vi "GUI_Syringe_Pump.vi"() -> ()   [LabVIEW 2020]
uses:
  <vilib>/Instr/_visa.llb/VISA Configure Serial Port (Instr).vi
panel:
  in  "Reset4":bool
  in  "Reset3":bool
  in  "Reset2":bool
  out "Remains4":string
  out "Remains3":string
  out "Remains2":string
  out "Dispensed4":string
  out "Dispensed3":string
  out "Dispensed2":string
  in  "Pump4\nStart/Stop":bool
  in  "Pump3\nStart/Stop":bool
  in  "Pump2\nStart/Stop":bool
  out "Diameter4 (mm)":dbl
  in  "dia4 (mm)":dbl=0.1 caption="Set Diameter (mm)" min=0.1 max=50.0
  in  "Syringe Selection4":string(combo)="CUS"
  out "Min rate4":dbl caption="Min rate" format="%#_4g"
  out "Max rate4":dbl format="%#_4g"
  in  "Direction4":string(combo)="inf"
  in  "Target Vol4":dbl caption="Target Vol (ul)"
  in  "Units4":string(combo)="mm"
  in  "Set rate4":dbl format="%#_4g"
  out "Diameter3 (mm)":dbl
  in  "dia3 (mm)":dbl=0.1 caption="Set Diameter (mm)" min=0.1 max=50.0
  in  "Syringe Selection3":string(combo)="CUS"
  out "Min rate3":dbl caption="Min rate" format="%#_4g"
  out "Max rate3":dbl format="%#_4g"
  in  "Direction3":string(combo)="inf"
  in  "Target Vol3":dbl caption="Target Vol (ul)"
  in  "Units3":string(combo)="mm"
  in  "Set rate3":dbl format="%#_4g"
  out "Diameter2 (mm)":dbl
  in  "dia2 (mm)":dbl=0.1 caption="Set Diameter (mm)" min=0.1 max=50.0
  in  "Syringe Selection2":string(combo)="BDP1MM"
  out "Min rate2":dbl caption="Min rate" format="%#_4g"
  out "Max rate2":dbl format="%#_4g"
  in  "Direction2":string(combo)="inf"
  in  "Target Vol2":dbl=1234.0 caption="Target Vol (ul)"
  in  "Units2":string(combo)="uh"
  in  "Set rate2":dbl=1000.0 format="%#_4g"
  out "Diameter1 (mm)":dbl
  in  "Syringe Selection1":string(combo)="BDP1MM"
  out "Remains1":string
  in  "Reset1":bool
  out "Dispensed1":string
  out "Baud Rate":string
  in  "Communication\nOn/Off":bool=TRUE
  in  "Pump1\nStart/Stop":bool
  out "Min rate1":dbl caption="Min rate" format="%#_4g"
  out "Max rate1":dbl format="%#_4g"
  in  "Send1":bool
  in  "Direction1":string(combo)="inf"
  in  "Target Vol1":dbl=1000.0 caption="Target Vol (ul)"
  in  "Units1":string(combo)="uh"
  in  "Set rate1":dbl=123.0 format="%#_4g"
  in  "dia1 (mm)":dbl=0.1 caption="Set Diameter (mm)" min=0.1 max=50.0
  in  "COM port number":refnum<visa-resource-name>
  # "Communication Setting"
  # "Cockpit"
  # "Pump1"
  # "Pump3"
  # "Pump4"
  # "Pump2"
  # "[Pump1] Syringe Setting"
  # "[Pump2] Syringe Setting"
  # "[Pump3] Syringe Setting"
  # "[Pump4] Syringe Setting"
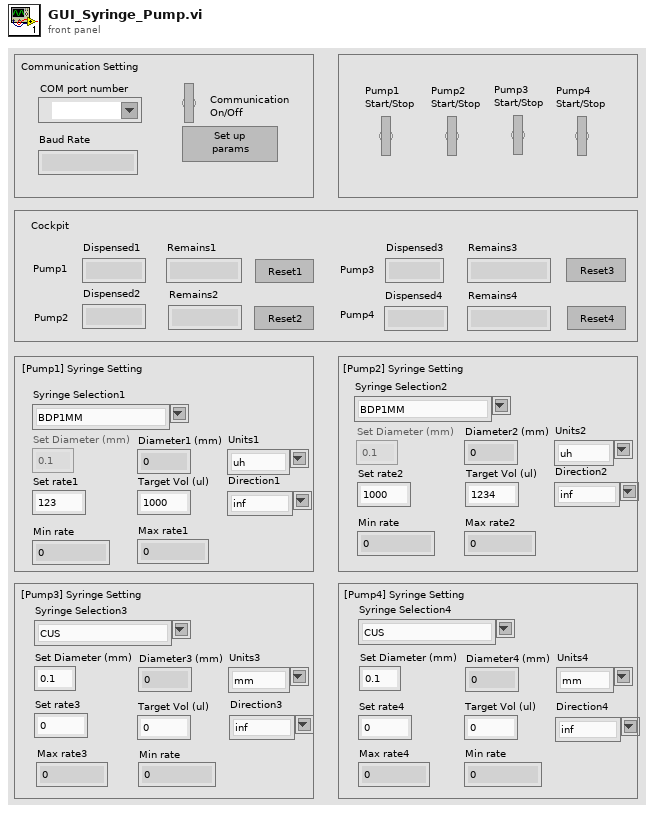
[diagram p1: front panel]
types:
  T1 = enum8{"Enabled", "Disabled", "Disabled and Grayed Out"}
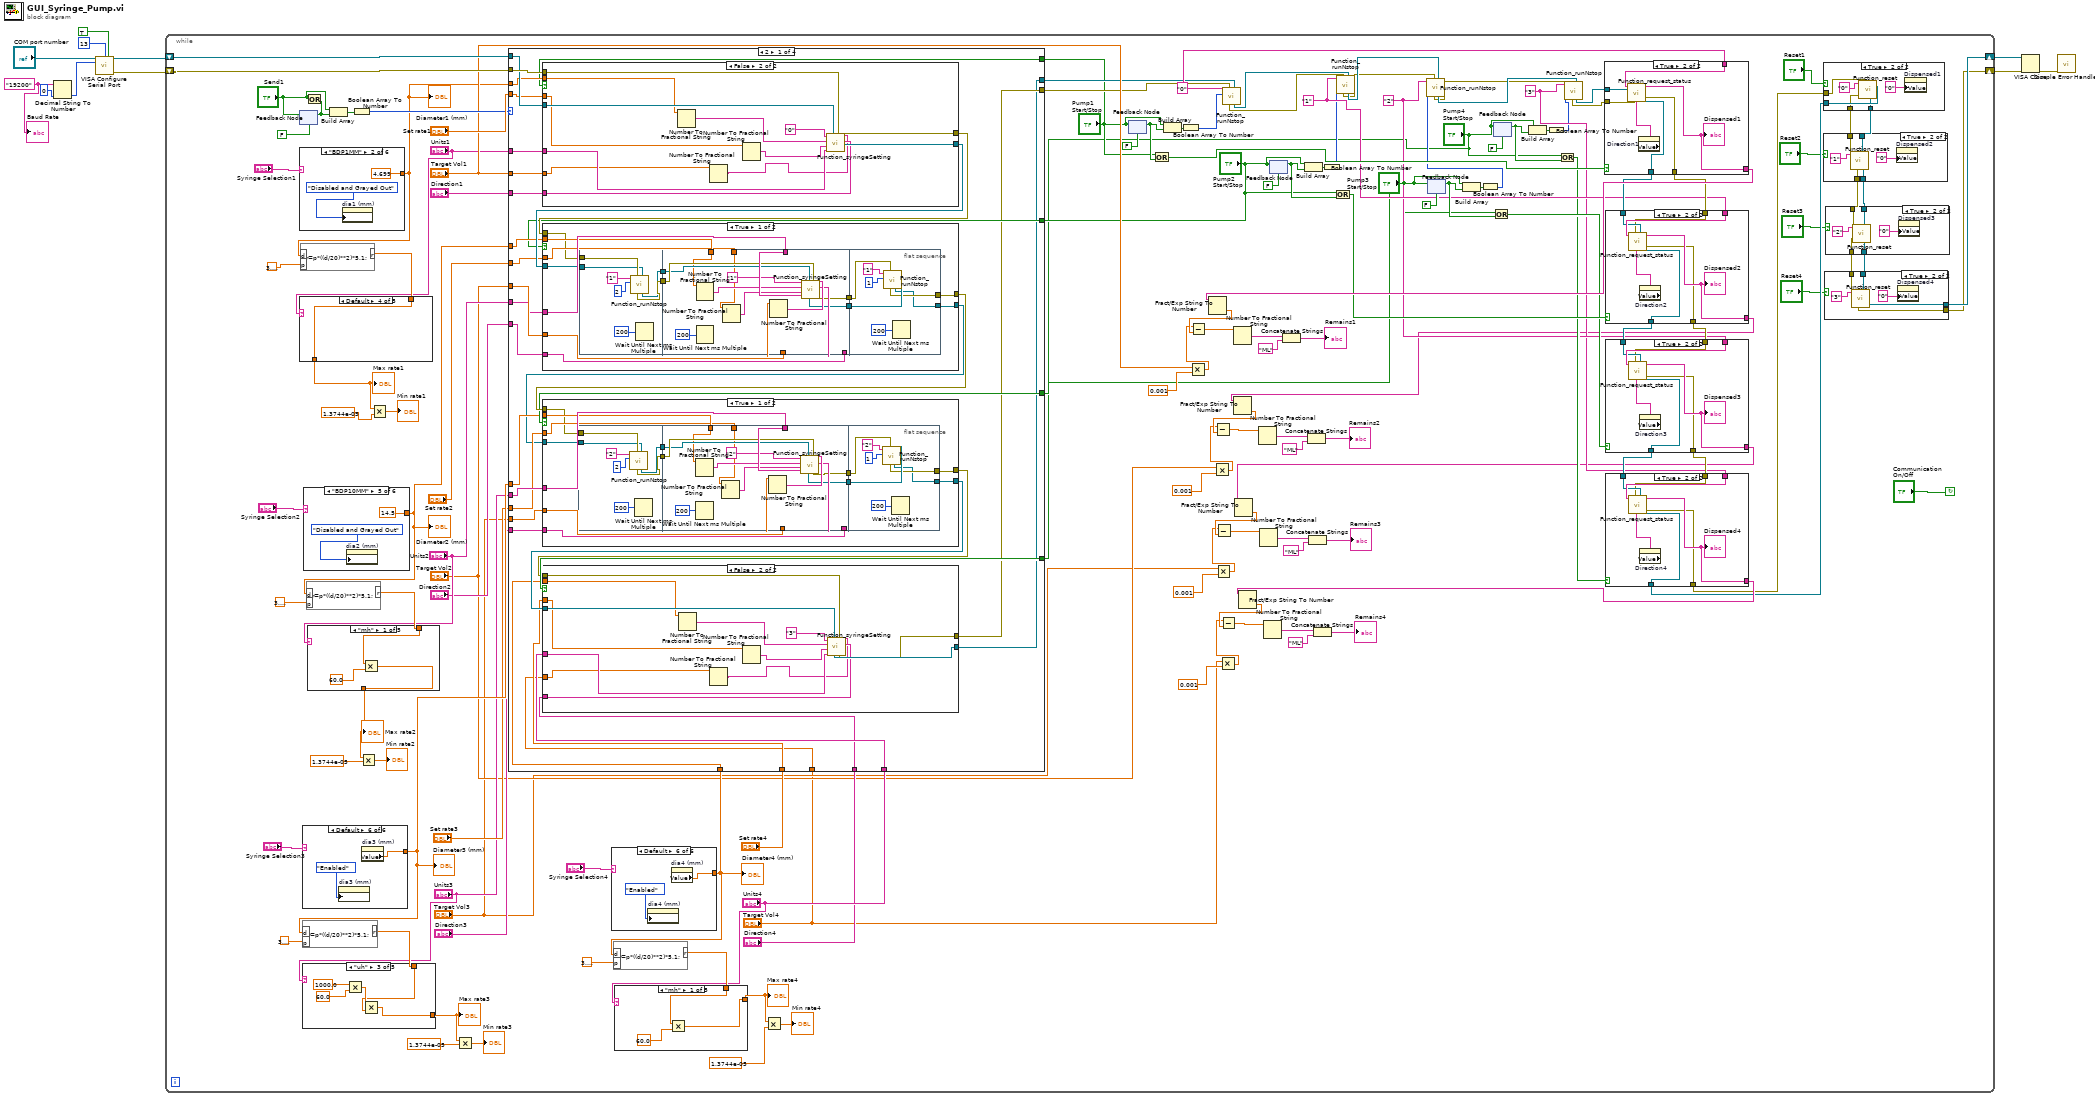
[diagram p0: block diagram]
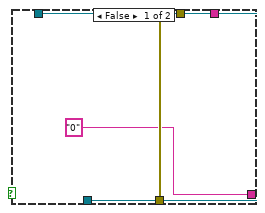
[diagram p6: hidden frame]
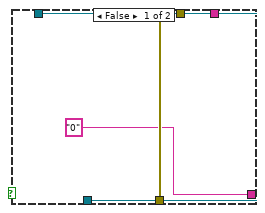
[diagram p7: hidden frame]
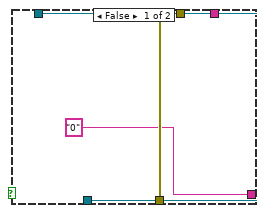
[diagram p8: hidden frame]
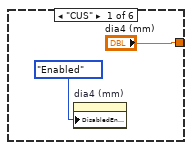
[diagram p9: hidden frame]
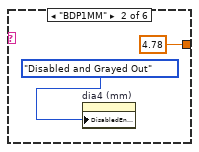
[diagram p10: hidden frame]
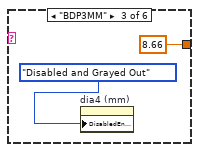
[diagram p11: hidden frame]
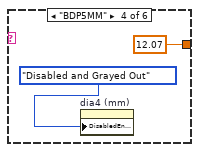
[diagram p12: hidden frame]
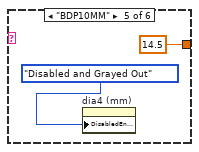
[diagram p13: hidden frame]
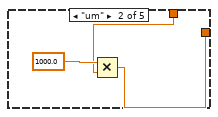
[diagram p14: hidden frame]
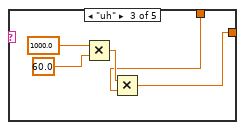
[diagram p15: hidden frame]
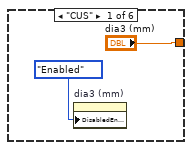
[diagram p18: hidden frame]
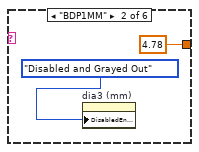
[diagram p19: hidden frame]
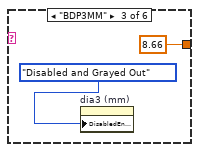
[diagram p20: hidden frame]
diagram:
  w1 = "19200" ("Baud Rate")
  n1 = Decimal String To Number(string=w1, default (0L)=u32 0 ("default (0 I32)")) -> (number=w9:u32)  [unwired: 1 in, 1 out]
  n2 = call-poly "VISA Configure Serial Port"("VISA resource name"="COM port number", "termination char\n(0xA = '\\n' = LF)"=u8 13 ("termination char\n(0xA = '\\n' = LF)"), "Enable Termination\nChar (T)"=TRUE ("Enable Termination\nChar (T)"), "baud rate (9600)"=w9) -> ("VISA resource name out"=w6:refnum<visa-resource-name>, "error out"=w5:errorcluster)  [unwired: 10 in]
  n3 = while {
    shift-right: [w23] -> w4
    shift-left: w6 -> [w152]
    shift-right: [w22] -> w3
    shift-left: w5 -> [w151]
    stop <- "Communication\nOn/Off" continue-if-true
    w63 = "3" ("trimmed string")
    w64 = "2" ("trimmed string")
    w72 = "1" ("trimmed string")
    w92 = "0" ("trimmed string")
    n4 = case shown="\"BDP1MM\"" "Syringe Selection1" {
      tunnel: ["dia1 (mm)" 4.699 ("dia (mm)") 8.66 ("dia (mm)") 12.07 ("dia (mm)") 14.5 ("dia (mm)") w302] -> w124
      frame "CUS" {
        n5 = property on="dia1 (mm)" class="DigNum (strict)"("DisabledEnum"=T1."Enabled" ("Disabled")) -> ()  [unwired: 2 in, 2 out]
      }
      frame "BDP1MM" {
        n6 = property on="dia1 (mm)" class="DigNum (strict)"("DisabledEnum"=T1."Disabled and Grayed Out" ("Disabled")) -> ()  [unwired: 2 in, 2 out]
      }
      frame "BDP3MM" {
        n7 = property on="dia1 (mm)" class="DigNum (strict)"("DisabledEnum"=T1."Disabled and Grayed Out" ("Disabled")) -> ()  [unwired: 2 in, 2 out]
      }
      frame "BDP5MM" {
        n8 = property on="dia1 (mm)" class="DigNum (strict)"("DisabledEnum"=T1."Disabled and Grayed Out" ("Disabled")) -> ()  [unwired: 2 in, 2 out]
      }
      frame "BDP10MM" {
        n9 = property on="dia1 (mm)" class="DigNum (strict)"("DisabledEnum"=T1."Disabled and Grayed Out" ("Disabled")) -> ()  [unwired: 2 in, 2 out]
      }
      frame Default {
        n10 = property on="dia1 (mm)" class="DigNum (strict)"("DisabledEnum"=T1."Enabled" ("Disabled")) -> ()  [unwired: 2 in, 2 out]
        n11 = property on="dia1 (mm)" class="DigNum (strict)"() -> ("Value"=w302:dbl)  [unwired: 2 in, 2 out]
      }
    }
    "Diameter1 (mm)" <- w124
    n12 = feedback #1(FALSE ("Go 1")) -> (w138:bool)
    n13 = feedback-in #1("Send1") -> ()
    n14 = formula code="r=p*((d/20)**2)*5.1;"("d"=w124, "p"=3.141592653589793) -> ("r"=w144:dbl)
    n15 = case shown="Default" "Units1" {
      tunnel: w144 -> [w314 w316 w320 w324 w325]
      tunnel: [w313 w317 w319 w324 w325] -> w145
      frame "mh" {
        n16 = Multiply(x=w314, y=60.0) -> (x*y=w313:dbl)
      }
      frame "um" {
        n17 = Multiply(x=1000.0, y=w316) -> (x*y=w317:dbl)
      }
      frame "uh" {
        n18 = Multiply(x=1000.0, y=60.0) -> (x*y=w323:dbl)
        n19 = Multiply(x=w323, y=w320) -> (x*y=w319:dbl)
      }
      frame Default {
      }
      frame "mm" {
      }
    }
    "Max rate1" <- w145
    n20 = case shown="Default" "Syringe Selection3" {
      tunnel: ["dia3 (mm)" 4.78 ("dia (mm)") 8.66 ("dia (mm)") 12.07 ("dia (mm)") 14.5 ("dia (mm)") w252] -> w106
      frame "CUS" {
        n21 = property on="dia3 (mm)" class="DigNum (strict)"("DisabledEnum"=T1."Enabled" ("Disabled")) -> ()  [unwired: 2 in, 2 out]
      }
      frame "BDP1MM" {
        n22 = property on="dia3 (mm)" class="DigNum (strict)"("DisabledEnum"=T1."Disabled and Grayed Out" ("Disabled")) -> ()  [unwired: 2 in, 2 out]
      }
      frame "BDP3MM" {
        n23 = property on="dia3 (mm)" class="DigNum (strict)"("DisabledEnum"=T1."Disabled and Grayed Out" ("Disabled")) -> ()  [unwired: 2 in, 2 out]
      }
      frame "BDP5MM" {
        n24 = property on="dia3 (mm)" class="DigNum (strict)"("DisabledEnum"=T1."Disabled and Grayed Out" ("Disabled")) -> ()  [unwired: 2 in, 2 out]
      }
      frame "BDP10MM" {
        n25 = property on="dia3 (mm)" class="DigNum (strict)"("DisabledEnum"=T1."Disabled and Grayed Out" ("Disabled")) -> ()  [unwired: 2 in, 2 out]
      }
      frame Default {
        n26 = property on="dia3 (mm)" class="DigNum (strict)"("DisabledEnum"=T1."Enabled" ("Disabled")) -> ()  [unwired: 2 in, 2 out]
        n27 = property on="dia3 (mm)" class="DigNum (strict)"() -> ("Value"=w252:dbl)  [unwired: 2 in, 2 out]
      }
    }
    "Diameter3 (mm)" <- w106
    n28 = formula code="r=p*((d/20)**2)*5.1;"("d"=w106, "p"=3.141592653589793) -> ("r"=w108:dbl)
    n29 = case shown="\"uh\"" "Units3" {
      tunnel: w108 -> [w254 w256 w260 w264 w265]
      tunnel: [w253 w257 w259 w264 w265] -> w109
      frame "mh" {
        n30 = Multiply(x=w254, y=60.0) -> (x*y=w253:dbl)
      }
      frame "um" {
        n31 = Multiply(x=1000.0, y=w256) -> (x*y=w257:dbl)
      }
      frame "uh" {
        n32 = Multiply(x=1000.0, y=60.0) -> (x*y=w263:dbl)
        n33 = Multiply(x=w263, y=w260) -> (x*y=w259:dbl)
      }
      frame Default {
      }
      frame "mm" {
      }
    }
    "Max rate3" <- w109
    n34 = case shown="\"BDP10MM\"" "Syringe Selection2" {
      tunnel: ["dia2 (mm)" 4.78 ("dia (mm)") 8.66 ("dia (mm)") 12.07 ("dia (mm)") 14.5 ("dia (mm)") w277] -> w116
      frame "CUS" {
        n35 = property on="dia2 (mm)" class="DigNum (strict)"("DisabledEnum"=T1."Enabled" ("Disabled")) -> ()  [unwired: 2 in, 2 out]
      }
      frame "BDP1MM" {
        n36 = property on="dia2 (mm)" class="DigNum (strict)"("DisabledEnum"=T1."Disabled and Grayed Out" ("Disabled")) -> ()  [unwired: 2 in, 2 out]
      }
      frame "BDP3MM" {
        n37 = property on="dia2 (mm)" class="DigNum (strict)"("DisabledEnum"=T1."Disabled and Grayed Out" ("Disabled")) -> ()  [unwired: 2 in, 2 out]
      }
      frame "BDP5MM" {
        n38 = property on="dia2 (mm)" class="DigNum (strict)"("DisabledEnum"=T1."Disabled and Grayed Out" ("Disabled")) -> ()  [unwired: 2 in, 2 out]
      }
      frame "BDP10MM" {
        n39 = property on="dia2 (mm)" class="DigNum (strict)"("DisabledEnum"=T1."Disabled and Grayed Out" ("Disabled")) -> ()  [unwired: 2 in, 2 out]
      }
      frame Default {
        n40 = property on="dia2 (mm)" class="DigNum (strict)"("DisabledEnum"=T1."Enabled" ("Disabled")) -> ()  [unwired: 2 in, 2 out]
        n41 = property on="dia2 (mm)" class="DigNum (strict)"() -> ("Value"=w277:dbl)  [unwired: 2 in, 2 out]
      }
    }
    "Diameter2 (mm)" <- w116
    n42 = Or(x="Send1", y=w138) -> ()  [unwired: 1 out]
    n43 = formula code="r=p*((d/20)**2)*5.1;"("d"=w116, "p"=3.141592653589793) -> ("r"=w118:dbl)
    n44 = case shown="\"mh\"" "Units2" {
      tunnel: w118 -> [w279 w281 w285 w289 w290]
      tunnel: [w278 w282 w284 w289 w290] -> w119
      frame "mh" {
        n45 = Multiply(x=w279, y=60.0) -> (x*y=w278:dbl)
      }
      frame "um" {
        n46 = Multiply(x=1000.0, y=w281) -> (x*y=w282:dbl)
      }
      frame "uh" {
        n47 = Multiply(x=1000.0, y=60.0) -> (x*y=w288:dbl)
        n48 = Multiply(x=w288, y=w285) -> (x*y=w284:dbl)
      }
      frame Default {
      }
      frame "mm" {
      }
    }
    "Max rate2" <- w119
    n49 = Build Array("Send1", w138) -> (w141:bool[])
    n50 = Boolean Array To Number(Boolean array=w141) -> (number=w139:u32)
    n51 = Multiply(x=w119, y=1.3744e-05) -> (x*y=→"Min rate2":dbl)
    n52 = Multiply(x=w145, y=1.3744e-05) -> (x*y=→"Min rate1":dbl)
    n53 = Multiply(x=w109, y=1.3744e-05) -> (x*y=→"Min rate3":dbl)
    n54 = case shown="Default" "Syringe Selection4" {
      tunnel: ["dia4 (mm)" 4.78 ("dia (mm)") 8.66 ("dia (mm)") 12.07 ("dia (mm)") 14.5 ("dia (mm)") w227] -> w96
      frame "CUS" {
        n55 = property on="dia4 (mm)" class="DigNum (strict)"("DisabledEnum"=T1."Enabled" ("Disabled")) -> ()  [unwired: 2 in, 2 out]
      }
      frame "BDP1MM" {
        n56 = property on="dia4 (mm)" class="DigNum (strict)"("DisabledEnum"=T1."Disabled and Grayed Out" ("Disabled")) -> ()  [unwired: 2 in, 2 out]
      }
      frame "BDP3MM" {
        n57 = property on="dia4 (mm)" class="DigNum (strict)"("DisabledEnum"=T1."Disabled and Grayed Out" ("Disabled")) -> ()  [unwired: 2 in, 2 out]
      }
      frame "BDP5MM" {
        n58 = property on="dia4 (mm)" class="DigNum (strict)"("DisabledEnum"=T1."Disabled and Grayed Out" ("Disabled")) -> ()  [unwired: 2 in, 2 out]
      }
      frame "BDP10MM" {
        n59 = property on="dia4 (mm)" class="DigNum (strict)"("DisabledEnum"=T1."Disabled and Grayed Out" ("Disabled")) -> ()  [unwired: 2 in, 2 out]
      }
      frame Default {
        n60 = property on="dia4 (mm)" class="DigNum (strict)"("DisabledEnum"=T1."Enabled" ("Disabled")) -> ()  [unwired: 2 in, 2 out]
        n61 = property on="dia4 (mm)" class="DigNum (strict)"() -> ("Value"=w227:dbl)  [unwired: 2 in, 2 out]
      }
    }
    "Diameter4 (mm)" <- w96
    n62 = case shown="2" w139 {
      tunnel: w152 -> [w357 w576 w579 w580]
      tunnel: w151 -> [w358 w577 w578 w581]
      tunnel: [w333 w577 w578 w581] -> w91
      tunnel: [w332 w576 w579 w580] -> w90
      tunnel: w124 -> [w354 _ _ _]
      tunnel: "Set rate1" -> [w353 _ _ _]
      tunnel: "Units1" -> [w356 _ _ _]
      tunnel: "Target Vol1" -> [w355 _ _ _]
      tunnel: "Direction1" -> [w359 _ _ _]
      tunnel: w116 -> [w346 _ _ _]
      tunnel: "Set rate2" -> [w347 _ _ _]
      tunnel: "Units2" -> [w348 _ _ _]
      tunnel: "Target Vol2" -> [w349 _ _ _]
      tunnel: "Direction2" -> [w350 _ _ _]
      tunnel: w106 -> [w338 _ _ _]
      tunnel: "Set rate3" -> [w339 _ _ _]
      tunnel: "Units3" -> [w340 _ _ _]
      tunnel: "Direction3" -> [w342 _ _ _]
      tunnel: "Target Vol3" -> [w341 _ _ _]
      tunnel: w96 -> [w330 _ _ _]
      tunnel: "Set rate4" -> [w329 _ _ _]
      tunnel: "Units4" -> [w328 _ _ _]
      tunnel: "Target Vol4" -> [w326 _ _ _]
      tunnel: "Direction4" -> [w327 _ _ _]
      tunnel: "Pump1\nStart/Stop" -> [w331 _ _ _]
      tunnel: "Pump2\nStart/Stop" -> [w345 _ _ _]
      tunnel: "Pump3\nStart/Stop" -> [w343 _ _ _]
      tunnel: "Pump4\nStart/Stop" -> [w336 _ _ _]
      frame 2 {
        n63 = case shown="False" w331 {
          tunnel: w359 -> [w534 w570]
          tunnel: w358 -> [w529 w575]
          tunnel: w357 -> [w528 w574]
          tunnel: w356 -> [w533 w571]
          tunnel: w355 -> [w532 w564]
          tunnel: w354 -> [w531 w568]
          tunnel: w353 -> [w530 w566]
          tunnel: [w522 w572] -> w352
          tunnel: [w523 w573] -> w351
          frame True {
            n64 = flat-sequence {
              tunnel: w529 -> [w541]
              tunnel: w528 -> [w540]
              tunnel: [w539] -> w527
              tunnel: [w538] -> w526
              tunnel: w534 -> [w554]
              tunnel: w533 -> [w553]
              tunnel: w532 -> [w551]
              tunnel: w531 -> [w547]
              tunnel: w530 -> [w545]
              tunnel: w527 -> [w543]
              tunnel: w526 -> [w550]
              tunnel: [w549] -> w525
              tunnel: [w542] -> w524
              tunnel: w525 -> [w562]
              tunnel: w524 -> [w561]
              tunnel: [w560] -> w522
              tunnel: [w559] -> w523
              frame #0 {
                n65 = call "Function_runNstop.vi"("VISA resource name in"=w540, "error in"=w541, "condition"=2, "Server addr"="0" ("trimmed string")) -> ("VISA resource name out"=w538:refnum<visa-resource-name>, "error out"=w539:errorcluster)  [unwired: 6 in]
                n66 = Wait Until Next ms Multiple(millisecond multiple=u32 200) -> ()  [unwired: 1 out]
              }
              frame #1 {
                n67 = Number To Fractional String(number=w547) -> (F-format string=w546:string)  [unwired: 3 in]
                n68 = Wait Until Next ms Multiple(millisecond multiple=u32 200) -> ()  [unwired: 1 out]
                n69 = Number To Fractional String(number=w545) -> (F-format string=w544:string)  [unwired: 3 in]
                n70 = Number To Fractional String(number=w551) -> (F-format string=w555:string)  [unwired: 3 in]
                n71 = call "Function_syringeSetting.vi"("Direction"=w554, "target volume- string"=w555, "error in"=w543, "VISA resource name in"=w550, "units"=w553, "set rate- string"=w544, "diameter(mm)-string"=w546, "address (string)"="0" ("Pump Add")) -> ("error out"=w549:errorcluster, "VISA resource name out"=w542:refnum<visa-resource-name>)  [unwired: 2 in]
              }
              frame #2 {
                n72 = call "Function_runNstop.vi"("VISA resource name in"=w561, "error in"=w562, "condition"=1, "Server addr"="0") -> ("VISA resource name out"=w559:refnum<visa-resource-name>, "error out"=w560:errorcluster)  [unwired: 6 in]
                n73 = Wait Until Next ms Multiple(millisecond multiple=u32 200) -> ()  [unwired: 1 out]
              }
            }
          }
          frame False {
            n74 = Number To Fractional String(number=w568) -> (F-format string=w567:string)  [unwired: 3 in]
            n75 = Number To Fractional String(number=w564) -> (F-format string=w563:string)  [unwired: 3 in]
            n76 = Number To Fractional String(number=w566) -> (F-format string=w565:string)  [unwired: 3 in]
            n77 = call "Function_syringeSetting.vi"("Direction"=w570, "target volume- string"=w563, "error in"=w575, "VISA resource name in"=w574, "units"=w571, "set rate- string"=w565, "diameter(mm)-string"=w567, "address (string)"="0" ("Pump Add")) -> ("error out"=w572:errorcluster, "VISA resource name out"=w573:refnum<visa-resource-name>)  [unwired: 2 in]
          }
        }
        n78 = case shown="True" w345 {
          tunnel: w350 -> [w480 w516]
          tunnel: w352 -> [w475 w521]
          tunnel: w351 -> [w474 w520]
          tunnel: w348 -> [w479 w517]
          tunnel: w349 -> [w478 w510]
          tunnel: w346 -> [w477 w514]
          tunnel: w347 -> [w476 w512]
          tunnel: [w468 w518] -> w344
          tunnel: [w469 w519] -> w337
          frame True {
            n79 = flat-sequence {
              tunnel: w475 -> [w487]
              tunnel: w474 -> [w486]
              tunnel: [w485] -> w473
              tunnel: [w484] -> w472
              tunnel: w480 -> [w500]
              tunnel: w479 -> [w499]
              tunnel: w478 -> [w497]
              tunnel: w477 -> [w491]
              tunnel: w476 -> [w489]
              tunnel: w473 -> [w496]
              tunnel: w472 -> [w495]
              tunnel: [w494] -> w471
              tunnel: [w493] -> w470
              tunnel: w471 -> [w508]
              tunnel: w470 -> [w507]
              tunnel: [w506] -> w468
              tunnel: [w505] -> w469
              frame #0 {
                n80 = call "Function_runNstop.vi"("VISA resource name in"=w486, "error in"=w487, "condition"=2, "Server addr"="1" ("trimmed string")) -> ("VISA resource name out"=w484:refnum<visa-resource-name>, "error out"=w485:errorcluster)  [unwired: 6 in]
                n81 = Wait Until Next ms Multiple(millisecond multiple=u32 200) -> ()  [unwired: 1 out]
              }
              frame #1 {
                n82 = Number To Fractional String(number=w491) -> (F-format string=w490:string)  [unwired: 3 in]
                n83 = Wait Until Next ms Multiple(millisecond multiple=u32 200) -> ()  [unwired: 1 out]
                n84 = Number To Fractional String(number=w489) -> (F-format string=w488:string)  [unwired: 3 in]
                n85 = Number To Fractional String(number=w497) -> (F-format string=w501:string)  [unwired: 3 in]
                n86 = call "Function_syringeSetting.vi"("Direction"=w500, "target volume- string"=w501, "error in"=w496, "VISA resource name in"=w495, "units"=w499, "set rate- string"=w488, "diameter(mm)-string"=w490, "address (string)"="1" ("Pump Add")) -> ("error out"=w494:errorcluster, "VISA resource name out"=w493:refnum<visa-resource-name>)  [unwired: 2 in]
              }
              frame #2 {
                n87 = call "Function_runNstop.vi"("VISA resource name in"=w507, "error in"=w508, "condition"=1, "Server addr"="1") -> ("VISA resource name out"=w505:refnum<visa-resource-name>, "error out"=w506:errorcluster)  [unwired: 6 in]
                n88 = Wait Until Next ms Multiple(millisecond multiple=u32 200) -> ()  [unwired: 1 out]
              }
            }
          }
          frame False {
            n89 = Number To Fractional String(number=w514) -> (F-format string=w513:string)  [unwired: 3 in]
            n90 = Number To Fractional String(number=w510) -> (F-format string=w509:string)  [unwired: 3 in]
            n91 = Number To Fractional String(number=w512) -> (F-format string=w511:string)  [unwired: 3 in]
            n92 = call "Function_syringeSetting.vi"("Direction"=w516, "target volume- string"=w509, "error in"=w521, "VISA resource name in"=w520, "units"=w517, "set rate- string"=w511, "diameter(mm)-string"=w513, "address (string)"="1" ("Pump Add")) -> ("error out"=w518:errorcluster, "VISA resource name out"=w519:refnum<visa-resource-name>)  [unwired: 2 in]
          }
        }
        n93 = case shown="True" w343 {
          tunnel: w342 -> [w426 w462]
          tunnel: w344 -> [w421 w467]
          tunnel: w337 -> [w414 w466]
          tunnel: w340 -> [w425 w463]
          tunnel: w341 -> [w424 w456]
          tunnel: w338 -> [w423 w460]
          tunnel: w339 -> [w422 w458]
          tunnel: [w415 w464] -> w335
          tunnel: [w416 w465] -> w334
          frame True {
            n94 = flat-sequence {
              tunnel: w421 -> [w433]
              tunnel: w414 -> [w432]
              tunnel: [w431] -> w420
              tunnel: [w430] -> w419
              tunnel: w426 -> [w446]
              tunnel: w425 -> [w445]
              tunnel: w424 -> [w443]
              tunnel: w423 -> [w437]
              tunnel: w422 -> [w435]
              tunnel: w420 -> [w442]
              tunnel: w419 -> [w441]
              tunnel: [w440] -> w418
              tunnel: [w439] -> w417
              tunnel: w418 -> [w454]
              tunnel: w417 -> [w453]
              tunnel: [w452] -> w415
              tunnel: [w451] -> w416
              frame #0 {
                n95 = call "Function_runNstop.vi"("VISA resource name in"=w432, "error in"=w433, "condition"=2, "Server addr"="2" ("trimmed string")) -> ("VISA resource name out"=w430:refnum<visa-resource-name>, "error out"=w431:errorcluster)  [unwired: 6 in]
                n96 = Wait Until Next ms Multiple(millisecond multiple=u32 200) -> ()  [unwired: 1 out]
              }
              frame #1 {
                n97 = Number To Fractional String(number=w437) -> (F-format string=w436:string)  [unwired: 3 in]
                n98 = Wait Until Next ms Multiple(millisecond multiple=u32 200) -> ()  [unwired: 1 out]
                n99 = Number To Fractional String(number=w435) -> (F-format string=w434:string)  [unwired: 3 in]
                n100 = Number To Fractional String(number=w443) -> (F-format string=w447:string)  [unwired: 3 in]
                n101 = call "Function_syringeSetting.vi"("Direction"=w446, "target volume- string"=w447, "error in"=w442, "VISA resource name in"=w441, "units"=w445, "set rate- string"=w434, "diameter(mm)-string"=w436, "address (string)"="2" ("Pump Add")) -> ("error out"=w440:errorcluster, "VISA resource name out"=w439:refnum<visa-resource-name>)  [unwired: 2 in]
              }
              frame #2 {
                n102 = call "Function_runNstop.vi"("VISA resource name in"=w453, "error in"=w454, "condition"=1, "Server addr"="2") -> ("VISA resource name out"=w451:refnum<visa-resource-name>, "error out"=w452:errorcluster)  [unwired: 6 in]
                n103 = Wait Until Next ms Multiple(millisecond multiple=u32 200) -> ()  [unwired: 1 out]
              }
            }
          }
          frame False {
            n104 = Number To Fractional String(number=w460) -> (F-format string=w459:string)  [unwired: 3 in]
            n105 = Number To Fractional String(number=w456) -> (F-format string=w455:string)  [unwired: 3 in]
            n106 = Number To Fractional String(number=w458) -> (F-format string=w457:string)  [unwired: 3 in]
            n107 = call "Function_syringeSetting.vi"("Direction"=w462, "target volume- string"=w455, "error in"=w467, "VISA resource name in"=w466, "units"=w463, "set rate- string"=w457, "diameter(mm)-string"=w459, "address (string)"="2" ("Pump Add")) -> ("error out"=w464:errorcluster, "VISA resource name out"=w465:refnum<visa-resource-name>)  [unwired: 2 in]
          }
        }
        n108 = case shown="False" w336 {
          tunnel: w327 -> [w372 w408]
          tunnel: w335 -> [w367 w413]
          tunnel: w334 -> [w360 w412]
          tunnel: w328 -> [w371 w409]
          tunnel: w326 -> [w370 w403]
          tunnel: w330 -> [w369 w406]
          tunnel: w329 -> [w368 w405]
          tunnel: [w361 w410] -> w333
          tunnel: [w362 w411] -> w332
          frame True {
            n109 = flat-sequence {
              tunnel: w367 -> [w379]
              tunnel: w360 -> [w378]
              tunnel: [w377] -> w366
              tunnel: [w376] -> w365
              tunnel: w372 -> [w392]
              tunnel: w371 -> [w391]
              tunnel: w370 -> [w389]
              tunnel: w369 -> [w383]
              tunnel: w368 -> [w381]
              tunnel: w366 -> [w388]
              tunnel: w365 -> [w387]
              tunnel: [w386] -> w364
              tunnel: [w385] -> w363
              tunnel: w364 -> [w400]
              tunnel: w363 -> [w399]
              tunnel: [w398] -> w361
              tunnel: [w397] -> w362
              frame #0 {
                n110 = call "Function_runNstop.vi"("VISA resource name in"=w378, "error in"=w379, "condition"=2, "Server addr"="3" ("trimmed string")) -> ("VISA resource name out"=w376:refnum<visa-resource-name>, "error out"=w377:errorcluster)  [unwired: 6 in]
                n111 = Wait Until Next ms Multiple(millisecond multiple=u32 200) -> ()  [unwired: 1 out]
              }
              frame #1 {
                n112 = Number To Fractional String(number=w383) -> (F-format string=w382:string)  [unwired: 3 in]
                n113 = Wait Until Next ms Multiple(millisecond multiple=u32 200) -> ()  [unwired: 1 out]
                n114 = Number To Fractional String(number=w381) -> (F-format string=w380:string)  [unwired: 3 in]
                n115 = Number To Fractional String(number=w389) -> (F-format string=w393:string)  [unwired: 3 in]
                n116 = call "Function_syringeSetting.vi"("Direction"=w392, "target volume- string"=w393, "error in"=w388, "VISA resource name in"=w387, "units"=w391, "set rate- string"=w380, "diameter(mm)-string"=w382, "address (string)"="3" ("Pump Add")) -> ("error out"=w386:errorcluster, "VISA resource name out"=w385:refnum<visa-resource-name>)  [unwired: 2 in]
              }
              frame #2 {
                n117 = call "Function_runNstop.vi"("VISA resource name in"=w399, "error in"=w400, "condition"=1, "Server addr"="3") -> ("VISA resource name out"=w397:refnum<visa-resource-name>, "error out"=w398:errorcluster)  [unwired: 6 in]
                n118 = Wait Until Next ms Multiple(millisecond multiple=u32 200) -> ()  [unwired: 1 out]
              }
            }
          }
          frame False {
            n119 = Number To Fractional String(number=w406) -> (F-format string=w401:string)  [unwired: 3 in]
            n120 = Number To Fractional String(number=w403) -> (F-format string=w402:string)  [unwired: 3 in]
            n121 = Number To Fractional String(number=w405) -> (F-format string=w404:string)  [unwired: 3 in]
            n122 = call "Function_syringeSetting.vi"("Direction"=w408, "target volume- string"=w402, "error in"=w413, "VISA resource name in"=w412, "units"=w409, "set rate- string"=w404, "diameter(mm)-string"=w401, "address (string)"="3" ("Pump Add")) -> ("error out"=w410:errorcluster, "VISA resource name out"=w411:refnum<visa-resource-name>)  [unwired: 2 in]
          }
        }
      }
      frame 1 {
      }
      frame Default {
      }
      frame 3 {
      }
    }
    n123 = formula code="r=p*((d/20)**2)*5.1;"("d"=w96, "p"=3.141592653589793) -> ("r"=w98:dbl)
    n124 = case shown="\"mh\"" "Units4" {
      tunnel: w98 -> [w229 w231 w235 w239 w240]
      tunnel: [w228 w232 w234 w239 w240] -> w99
      frame "mh" {
        n125 = Multiply(x=w229, y=60.0) -> (x*y=w228:dbl)
      }
      frame "um" {
        n126 = Multiply(x=1000.0, y=w231) -> (x*y=w232:dbl)
      }
      frame "uh" {
        n127 = Multiply(x=1000.0, y=60.0) -> (x*y=w238:dbl)
        n128 = Multiply(x=w238, y=w235) -> (x*y=w234:dbl)
      }
      frame Default {
      }
      frame "mm" {
      }
    }
    "Max rate4" <- w99
    n129 = Multiply(x=w99, y=1.3744e-05) -> (x*y=→"Min rate4":dbl)
    n130 = feedback #2(FALSE ("Motor Start/Stop")) -> (w136:bool)
    n131 = feedback-in #2("Pump1\nStart/Stop") -> ()
    n132 = Or(x="Pump1\nStart/Stop", y=w136) -> (x .or. y?=w135:bool)
    n133 = Build Array("Pump1\nStart/Stop", w136) -> (w153:bool[])
    n134 = Boolean Array To Number(Boolean array=w153) -> (number=w21:u32)
    n135 = Multiply(x="Target Vol1", y=0.001) -> (x*y=w129:dbl)
    n136 = Multiply(x="Target Vol2", y=0.001) -> (x*y=w59:dbl)
    n137 = Multiply(x="Target Vol3", y=0.001) -> (x*y=w52:dbl)
    n138 = Multiply(x="Target Vol4", y=0.001) -> (x*y=w45:dbl)
    n139 = call "Function_runNstop.vi"("VISA resource name in"=w90, "error in"=w91, "condition"=w21, "Server addr"=w92) -> ("VISA resource name out"=w86:refnum<visa-resource-name>, "error out"=w85:errorcluster)  [unwired: 6 in]
    n140 = feedback #3(FALSE ("Motor Start/Stop")) -> (w87:bool)
    n141 = feedback-in #3("Pump2\nStart/Stop") -> ()
    n142 = Build Array("Pump2\nStart/Stop", w87) -> (w89:bool[])
    n143 = Boolean Array To Number(Boolean array=w89) -> (number=w20:u32)
    n144 = Or(x="Pump2\nStart/Stop", y=w87) -> (x .or. y?=w69:bool)
    n145 = call "Function_runNstop.vi"("VISA resource name in"=w86, "error in"=w85, "condition"=w20, "Server addr"=w72) -> ("VISA resource name out"=w78:refnum<visa-resource-name>, "error out"=w13:errorcluster)  [unwired: 6 in]
    n146 = feedback #4(FALSE ("Motor Start/Stop")) -> (w82:bool)
    n147 = feedback-in #4("Pump3\nStart/Stop") -> ()
    n148 = Build Array("Pump3\nStart/Stop", w82) -> (w84:bool[])
    n149 = Boolean Array To Number(Boolean array=w84) -> (number=w19:u32)
    n150 = call "Function_runNstop.vi"("VISA resource name in"=w78, "error in"=w13, "condition"=w19, "Server addr"=w64) -> ("VISA resource name out"=w77:refnum<visa-resource-name>, "error out"=w12:errorcluster)  [unwired: 6 in]
    n151 = Or(x="Pump3\nStart/Stop", y=w82) -> (x .or. y?=w68:bool)
    n152 = feedback #5(FALSE ("Motor Start/Stop")) -> (w79:bool)
    n153 = feedback-in #5("Pump4\nStart/Stop") -> ()
    n154 = Build Array("Pump4\nStart/Stop", w79) -> (w81:bool[])
    n155 = Boolean Array To Number(Boolean array=w81) -> (number=w18:u32)
    n156 = Or(x="Pump4\nStart/Stop", y=w79) -> (x .or. y?=w67:bool)
    n157 = call "Function_runNstop.vi"("VISA resource name in"=w77, "error in"=w12, "condition"=w18, "Server addr"=w63) -> ("VISA resource name out"=w76:refnum<visa-resource-name>, "error out"=w75:errorcluster)  [unwired: 6 in]
    n158 = case shown="True" w135 {
      tunnel: [w305 w307] -> w74
      tunnel: [w304 w306] -> w73
      tunnel: w76 -> [w305 w310]
      tunnel: w75 -> [w304 w309]
      tunnel: w92 -> [_ w311]
      tunnel: ["0" ("Vol Infused") w308] -> w134
      frame False {
      }
      frame True {
        n159 = property on="Direction1" class="CmbBox"() -> ("Value"=w312:string)  [unwired: 2 in, 2 out]
        n160 = call "Function_request_status.vi"("VISA resource name in"=w310, "error in"=w309, "Direction"=w312, "Server addr"=w311) -> ("Dispensed1"=w308:string, "VISA resource name out"=w307:refnum<visa-resource-name>, "error out"=w306:errorcluster)  [unwired: 5 in]
        "Dispensed1" <- w308
      }
    }
    n161 = Fract/Exp String To Number(string=w134) -> (number=w133:dbl)  [unwired: 3 in, 1 out]
    n162 = Subtract(x=w129, y=w133) -> (x-y=w132:dbl)
    n163 = Number To Fractional String(number=w132) -> (F-format string=w128:string)  [unwired: 3 in]
    n164 = Concatenate Strings(w128, "ML" ("string")) -> (→"Remains1":string)
    n165 = case shown="True" w69 {
      tunnel: [w208 w210] -> w71
      tunnel: [w207 w209] -> w70
      tunnel: w74 -> [w208 w213]
      tunnel: w73 -> [w207 w212]
      tunnel: w72 -> [_ w214]
      tunnel: ["0" ("Vol Infused") w211] -> w38
      frame False {
      }
      frame True {
        n166 = property on="Direction2" class="CmbBox"() -> ("Value"=w215:string)  [unwired: 2 in, 2 out]
        n167 = call "Function_request_status.vi"("VISA resource name in"=w213, "error in"=w212, "Direction"=w215, "Server addr"=w214) -> ("Dispensed1"=w211:string, "VISA resource name out"=w210:refnum<visa-resource-name>, "error out"=w209:errorcluster)  [unwired: 5 in]
        "Dispensed2" <- w211
      }
    }
    n168 = Fract/Exp String To Number(string=w38) -> (number=w62:dbl)  [unwired: 3 in, 1 out]
    n169 = Subtract(x=w59, y=w62) -> (x-y=w61:dbl)
    n170 = Number To Fractional String(number=w61) -> (F-format string=w58:string)  [unwired: 3 in]
    n171 = Concatenate Strings(w58, "ML" ("string")) -> (→"Remains2":string)
    n172 = case shown="True" w68 {
      tunnel: [w198 w200] -> w66
      tunnel: [w197 w199] -> w65
      tunnel: w71 -> [w198 w203]
      tunnel: w70 -> [w197 w202]
      tunnel: w64 -> [_ w204]
      tunnel: ["0" ("Vol Infused") w201] -> w37
      frame False {
      }
      frame True {
        n173 = property on="Direction3" class="CmbBox"() -> ("Value"=w205:string)  [unwired: 2 in, 2 out]
        n174 = call "Function_request_status.vi"("VISA resource name in"=w203, "error in"=w202, "Direction"=w205, "Server addr"=w204) -> ("Dispensed1"=w201:string, "VISA resource name out"=w200:refnum<visa-resource-name>, "error out"=w199:errorcluster)  [unwired: 5 in]
        "Dispensed3" <- w201
      }
    }
    n175 = Fract/Exp String To Number(string=w37) -> (number=w55:dbl)  [unwired: 3 in, 1 out]
    n176 = Subtract(x=w52, y=w55) -> (x-y=w54:dbl)
    n177 = Number To Fractional String(number=w54) -> (F-format string=w51:string)  [unwired: 3 in]
    n178 = Concatenate Strings(w51, "ML" ("string")) -> (→"Remains3":string)
    n179 = case shown="True" w67 {
      tunnel: [w188 w190] -> w33
      tunnel: [w187 w189] -> w34
      tunnel: w66 -> [w188 w193]
      tunnel: w65 -> [w187 w192]
      tunnel: w63 -> [_ w194]
      tunnel: ["0" ("Vol Infused") w191] -> w36
      frame False {
      }
      frame True {
        n180 = property on="Direction4" class="CmbBox"() -> ("Value"=w195:string)  [unwired: 2 in, 2 out]
        n181 = call "Function_request_status.vi"("VISA resource name in"=w193, "error in"=w192, "Direction"=w195, "Server addr"=w194) -> ("Dispensed1"=w191:string, "VISA resource name out"=w190:refnum<visa-resource-name>, "error out"=w189:errorcluster)  [unwired: 5 in]
        "Dispensed4" <- w191
      }
    }
    n182 = Fract/Exp String To Number(string=w36) -> (number=w48:dbl)  [unwired: 3 in, 1 out]
    n183 = Subtract(x=w45, y=w48) -> (x-y=w47:dbl)
    n184 = Number To Fractional String(number=w47) -> (F-format string=w44:string)  [unwired: 3 in]
    n185 = Concatenate Strings(w44, "ML" ("string")) -> (→"Remains4":string)
    n186 = case shown="True" "Reset1" {
      tunnel: w34 -> [w178 w185]
      tunnel: w33 -> [w179 w184]
      tunnel: [w178 w181] -> w31
      tunnel: [w179 w180] -> w30
      frame False {
      }
      frame True {
        n187 = call "Function_reset.vi"("VISA resource name in"=w184, "error in"=w185, "Server addr"="0" ("trimmed string")) -> ("VISA resource name out"=w180:refnum<visa-resource-name>, "error out"=w181:errorcluster)  [unwired: 7 in]
        n188 = property on="Dispensed1" class="Str"("Value"="0" ("Vol Infused")) -> ()  [unwired: 2 in, 2 out]
      }
    }
    n189 = case shown="True" "Reset2" {
      tunnel: w31 -> [w170 w177]
      tunnel: w30 -> [w171 w176]
      tunnel: [w170 w173] -> w27
      tunnel: [w171 w172] -> w26
      frame False {
      }
      frame True {
        n190 = call "Function_reset.vi"("VISA resource name in"=w176, "error in"=w177, "Server addr"="1" ("trimmed string")) -> ("VISA resource name out"=w172:refnum<visa-resource-name>, "error out"=w173:errorcluster)  [unwired: 7 in]
        n191 = property on="Dispensed2" class="Str"("Value"="0" ("Vol Infused")) -> ()  [unwired: 2 in, 2 out]
      }
    }
    n192 = case shown="True" "Reset3" {
      tunnel: w27 -> [w163 w169]
      tunnel: w26 -> [w162 w164]
      tunnel: [w163 w166] -> w25
      tunnel: [w162 w165] -> w24
      frame False {
      }
      frame True {
        n193 = call "Function_reset.vi"("VISA resource name in"=w164, "error in"=w169, "Server addr"="2" ("trimmed string")) -> ("VISA resource name out"=w165:refnum<visa-resource-name>, "error out"=w166:errorcluster)  [unwired: 7 in]
        n194 = property on="Dispensed3" class="Str"("Value"="0" ("Vol Infused")) -> ()  [unwired: 2 in, 2 out]
      }
    }
    n195 = case shown="True" "Reset4" {
      tunnel: w25 -> [w154 w161]
      tunnel: w24 -> [w155 w160]
      tunnel: [w155 w157] -> w23
      tunnel: [w154 w156] -> w22
      frame False {
      }
      frame True {
        n196 = call "Function_reset.vi"("VISA resource name in"=w160, "error in"=w161, "Server addr"="3" ("trimmed string")) -> ("VISA resource name out"=w157:refnum<visa-resource-name>, "error out"=w156:errorcluster)  [unwired: 7 in]
        n197 = property on="Dispensed4" class="Str"("Value"="0" ("Vol Infused")) -> ()  [unwired: 2 in, 2 out]
      }
    }
  }
  n198 = VISA Close(VISA resource name=w4, error in (no error)=w3) -> (error out=w2:errorcluster)
  n199 = call <vilib>:"Simple Error Handler.vi"("error in (no error)"=w2) -> ()  [unwired: 4 in, 5 out]
  "Baud Rate" <- w1
